vi "IsTagString.vi"(0 "Input String":string, 3 "Tag Desired":string="time=") -> (7 "Value String":string, 10 "Is Tag String":bool)   [LabVIEW 2013]
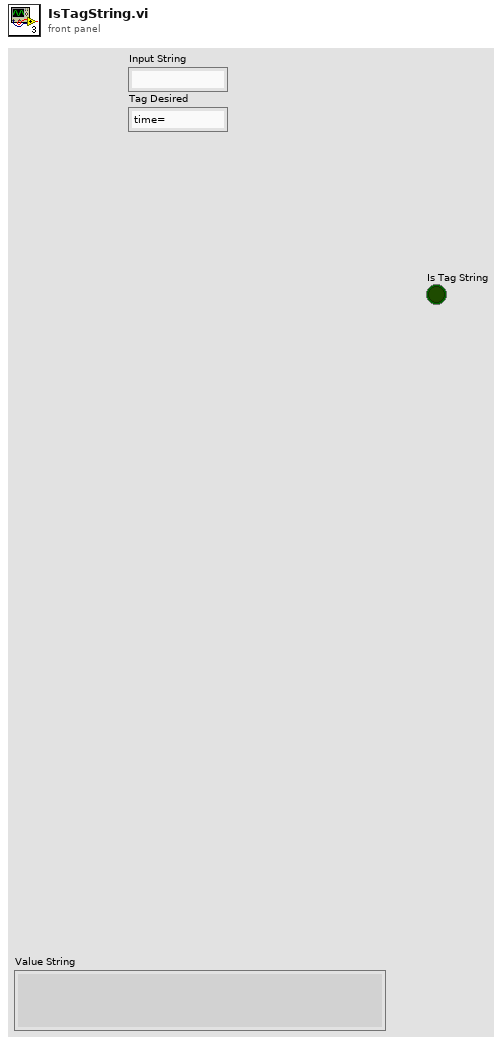
[diagram p1: front panel]
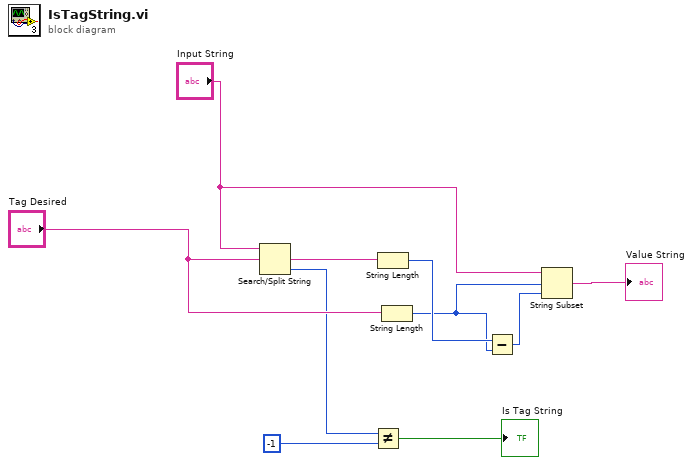
[diagram p0: block diagram]
diagram:
  n1 = Search/Split String(string="Input String", search string/char (-)="Tag Desired") -> (match + rest of string=w10:string, offset of match=w5:i32)  [unwired: 1 in, 1 out]
  n2 = Not Equal?(x=w5, y=-1) -> (x != y?=→"Is Tag String":bool)
  n3 = String Length(string=w10) -> (length=w8:i32)
  n4 = String Length(string="Tag Desired") -> (length=w7:i32)
  n5 = Subtract(x=w8, y=w7) -> (x-y=w6:i32)
  n6 = String Subset(string="Input String", offset (0)=w7, length (rest)=w6) -> (substring=→"Value String":string)
